vi "SDSU_ReadMux.vi"(7 "fd":i32, 8 "error in (no error)":errorcluster, 9 "argument":string, 10 "action":T3(ring), 11 "DACS":string[][](table)) -> (0 "error out":errorcluster, 1 "response":string, 2 "Table":string[][](table), 6 "fd out":i32)   [LabVIEW 2016]
panel:
  out "muxes out":T1(array[cluster])
  in  "muxes":T2
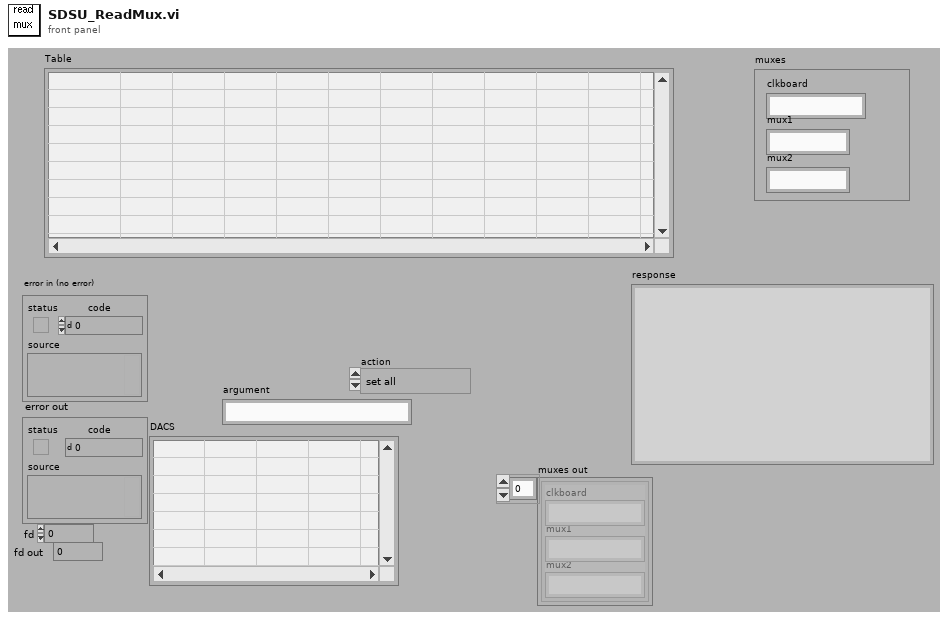
[diagram p1: front panel]
types:
  T1 = cluster{"clkboard":string, "mux1":string, "mux2":string}[]
  T2 = cluster{"clkboard":string, "mux1":string, "mux2":string}
  T3 = enum16{"set all", "set", "get all", "get list", "get"}
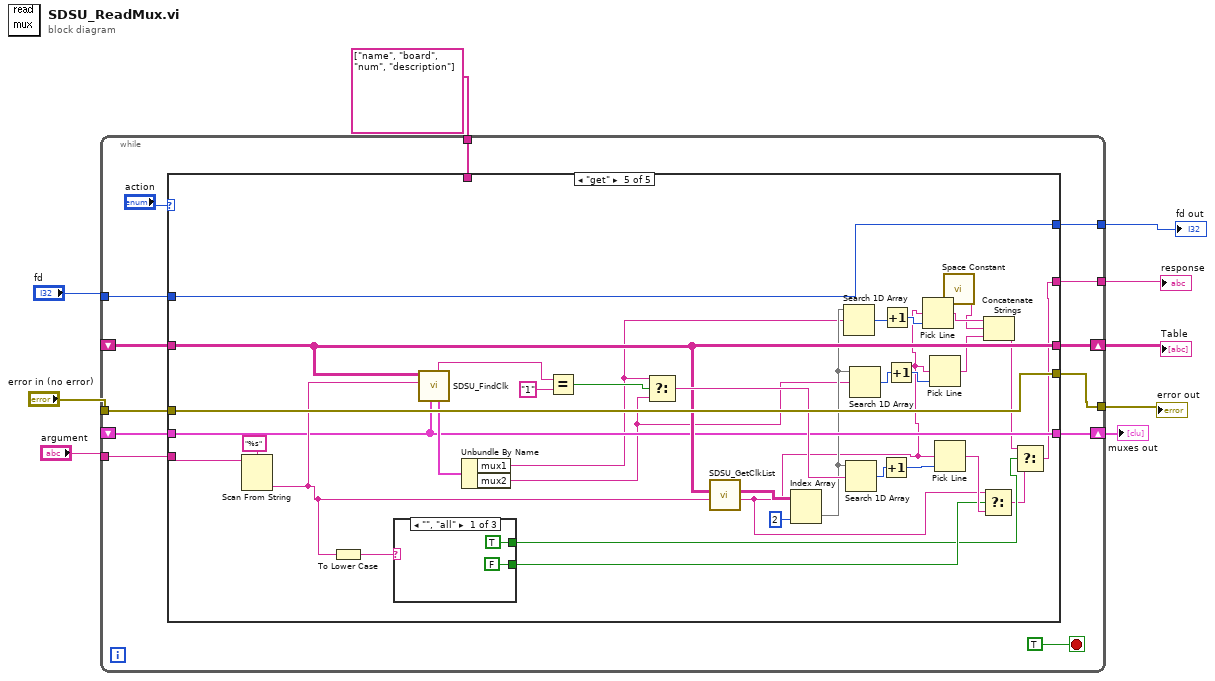
[diagram p0: block diagram]
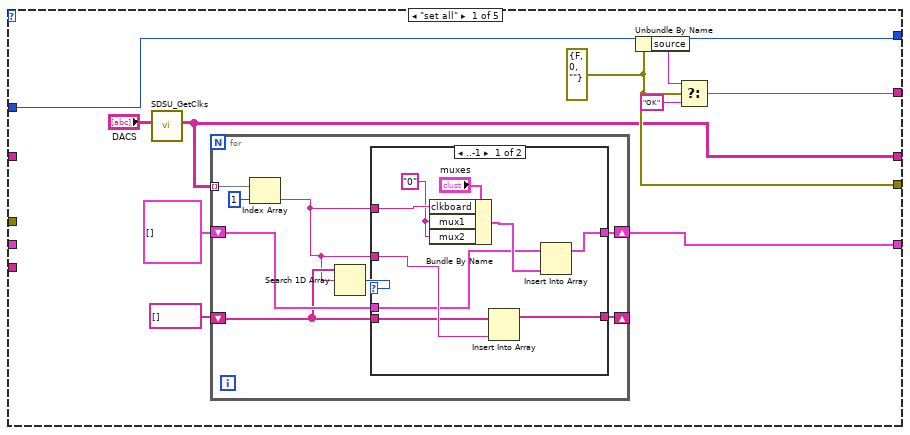
[diagram p2: hidden frame]
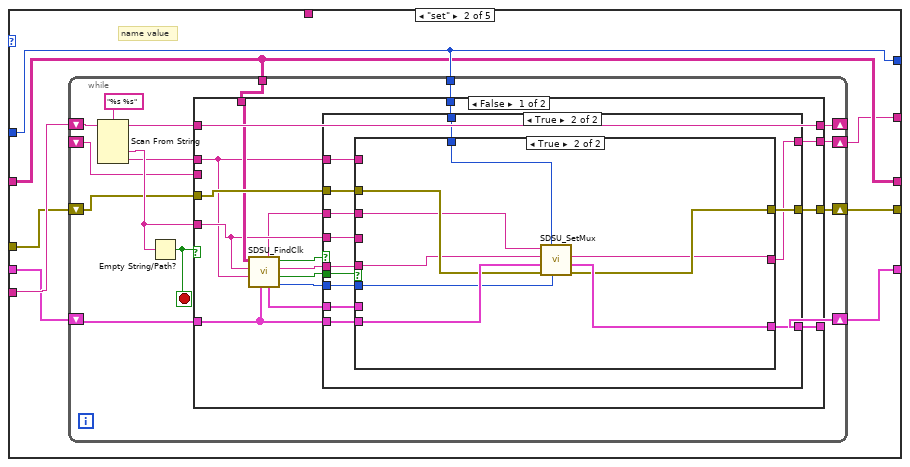
[diagram p4: hidden frame]
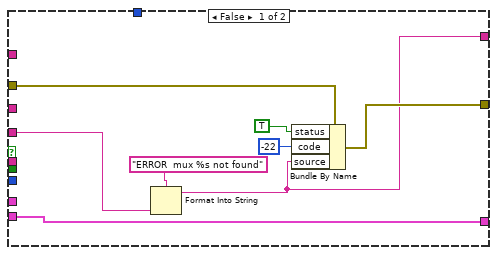
[diagram p5: hidden frame]
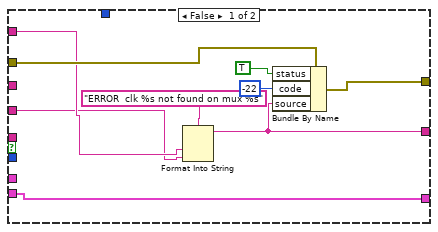
[diagram p6: hidden frame]
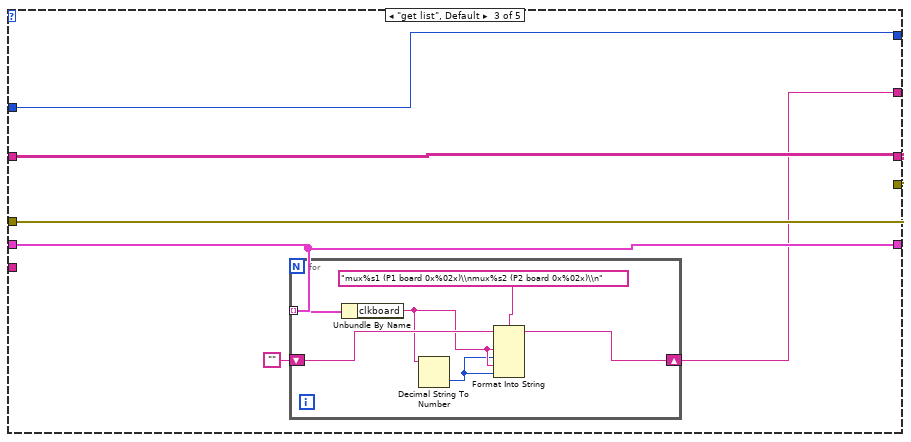
[diagram p8: hidden frame]
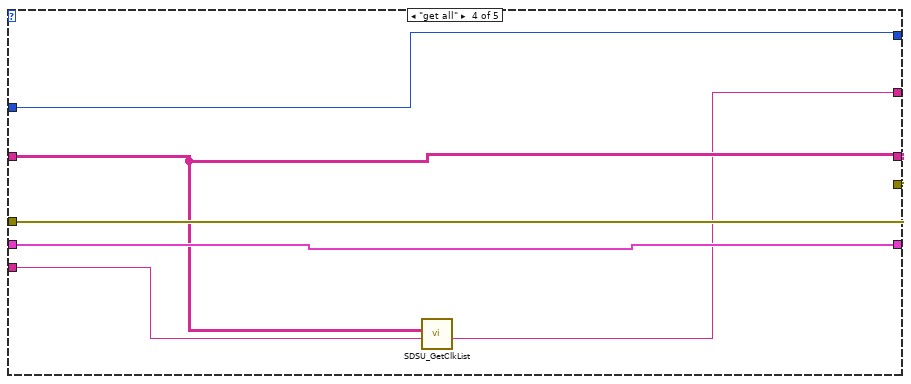
[diagram p9: hidden frame]
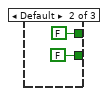
[diagram p10: hidden frame]
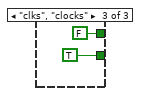
[diagram p11: hidden frame]
diagram:
  n1 = while {
    shift-right: [w21] -> w8
    shift-left: _ -> [w17]
    tunnel: "error in (no error)" -> [w20]
    tunnel: [w19] -> w2
    tunnel: [w10] -> w7
    tunnel: "argument" -> [w16]
    tunnel: "fd" -> [w15]
    tunnel: [w14] -> w4
    tunnel: string[] ["name", "board", "num", "description"] -> [w13]
    shift-right: [w12] -> w1
    shift-left: _ -> [w11]
    stop <- TRUE stop-if-true
    n2 = case shown="\"get\"" "action" {
      tunnel: [w27 w57 w137 w148 w168] -> w21
      tunnel: w20 -> [_ w53 w138 w150 w184]
      tunnel: [w28 w54 w138 w150 w184] -> w19
      tunnel: w17 -> [_ w57 w137 w148 w168]
      tunnel: w16 -> [_ w59 _ w147 w183]
      tunnel: w15 -> [w30 w58 w139 w151 w185]
      tunnel: [w30 w58 w139 w151 w185] -> w14
      tunnel: w13 -> [_ _ _ _ _]
      tunnel: [w26 w55 w136 w149 w167] -> w12
      tunnel: w11 -> [_ w56 w136 w149 w167]
      tunnel: [w23 w52 w134 w146 w152] -> w10
      frame "set all" {
        w28 = errorcluster {"status"=FALSE, "code"=0, "source"=""} ("input cluster")
        n3 = call "SDSU_GetClks.vi"("DACS"="DACS") -> ("Table"=w27:string[][])  [unwired: 10 out]
        n4 = for {
          tunnel: w27 -> [w40] mode=indexing
          shift-right: [w33] -> w26
          shift-left: T1 [] -> [w37]
          shift-right: [w36] -> _
          shift-left: string[] [] -> [w35]
          n5 = Index Array(array=w40, index=1) -> (element=w34:string)
          n6 = Search 1D Array(1D array=w35, element=w34) -> (index of element=w38:i32)  [unwired: 1 in]
          n7 = case shown="..-1" w38 {
            tunnel: w37 -> [w41 w50]
            tunnel: w34 -> [w49 _]
            tunnel: [w48 w51] -> w36
            tunnel: w35 -> [w47 w51]
            tunnel: w34 -> [w45 _]
            tunnel: [w42 w50] -> w33
            frame ..-1 {
              w44 = "0" ("element")
              n8 = Bundle By Name(cluster="muxes", "clkboard"=w45, "mux1"=w44, "mux2"=w44) -> (w43:T2)
              n9 = Insert Into Array(array=w47, new element=w49) -> (w48:string[])  [unwired: 1 in]
              n10 = Insert Into Array(array=w41, new element=w43) -> (w42:T1)  [unwired: 1 in]
            }
            frame Default {
            }
          }
        }
        n11 = Unbundle By Name(w28) -> ("source"=w32:string)
        n12 = Select(t=w32, s=w28, f="OK") -> (s? t:f=w23:string)
      }
      frame "set" {
        # "name value"
        n13 = while {
          shift-right: [w70] -> _
          shift-left: w59 -> [w73]
          tunnel: w58 -> [w67]
          tunnel: w57 -> [w66]
          shift-right: [w65] -> w55
          shift-left: w56 -> [w64]
          shift-right: [w63] -> w54
          shift-left: w53 -> [w62]
          shift-right: [w61] -> w52
          shift-left: _ -> [w60]
          stop <- w72 stop-if-true
          n14 = Scan From String(format string="%s %s", input string=w73) -> (remaining string=w71:string, output 1=w69:string, output 2=w68:string)  [unwired: 2 in, 4 out]
          n15 = Empty String/Path?(string/path=w69) -> (empty?=w72:bool)
          n16 = case shown="False" w72 {
            tunnel: w71 -> [w90 w133]
            tunnel: [w90 w133] -> w70
            tunnel: w69 -> [w84 _]
            tunnel: w62 -> [w89 w132]
            tunnel: w68 -> [w83 _]
            tunnel: [w88 w132] -> w63
            tunnel: [w87 w130] -> w61
            tunnel: w67 -> [w86 _]
            tunnel: w66 -> [w85 _]
            tunnel: w64 -> [w78 w131]
            tunnel: [w77 w131] -> w65
            tunnel: w60 -> [_ w130]
            frame False {
              n17 = call "SDSU_FindClk.vi"("muxes"=w78, "clk name"=w83, "mux name"=w84, "Table"=w85) -> ("mux index"=w75:i32, "found clk"=w81:bool, "clk num"=w80:string, "found mux"=w82:bool, "muxes out"=w79:T2, "mux num"=w76:string)  [unwired: 2 out]
              n18 = case shown="True" w82 {
                tunnel: w89 -> [w98 w110]
                tunnel: w84 -> [w94 w106]
                tunnel: [w93 w109] -> w88
                tunnel: [w92 w108] -> w87
                tunnel: w86 -> [_ w104]
                tunnel: w83 -> [_ w107]
                tunnel: w81 -> [_ w111]
                tunnel: w80 -> [_ w105]
                tunnel: w79 -> [_ w103]
                tunnel: w78 -> [w91 w102]
                tunnel: [w91 w100] -> w77
                tunnel: w76 -> [_ w101]
                tunnel: w75 -> [_ w99]
                frame False {
                  n19 = Format Into String(format string="ERROR  mux %s not found", w94) -> (resulting string=w92:string)  [unwired: 2 in, 1 out]
                  n20 = Bundle By Name(cluster=w98, "status"=TRUE, "code"=-22, "source"=w92) -> (w93:errorcluster)
                }
                frame True {
                  n21 = case shown="True" w111 {
                    tunnel: w110 -> [w118 w126]
                    tunnel: [w117 w127] -> w109
                    tunnel: [w116 w122] -> w108
                    tunnel: w107 -> [w113 _]
                    tunnel: w106 -> [w112 _]
                    tunnel: w105 -> [_ w124]
                    tunnel: w104 -> [_ w125]
                    tunnel: w103 -> [_ _]
                    tunnel: w102 -> [w114 w129]
                    tunnel: w101 -> [_ w121]
                    tunnel: [w114 w128] -> w100
                    tunnel: w99 -> [_ w123]
                    frame False {
                      n22 = Format Into String(format string="ERROR  clk %s not found on mux %s", w113, w112) -> (resulting string=w116:string)  [unwired: 2 in, 1 out]
                      n23 = Bundle By Name(cluster=w118, "status"=TRUE, "code"=-22, "source"=w116) -> (w117:errorcluster)
                    }
                    frame True {
                      n24 = call "SDSU_SetMux.vi"("muxes index"=w123, "fd"=w125, "error in (no error)"=w126, "muxes in"=w129, "clk"=w124, "mux"=w121) -> ("error IO"=w127:errorcluster, "muxes out"=w128:T1, "response"=w122:string)  [unwired: 3 out]
                    }
                  }
                }
              }
            }
            frame True {
            }
          }
        }
      }
      frame "get list", Default {
        n25 = for {
          tunnel: w136 -> [w142] mode=indexing
          shift-right: [w144] -> w134
          shift-left: "" -> [w143]
          n26 = Unbundle By Name(w142) -> ("clkboard"=w141:string)
          n27 = Decimal String To Number(string=w141) -> (number=w140:i32)  [unwired: 3 out]
          n28 = Format Into String(format string="mux%s1 (P1 board 0x%02x)\\nmux%s2 (P2 board 0x%02x)\\n", initial string=w143, w141, w140, w141, w140) -> (resulting string=w144:string)  [unwired: 1 in, 1 out]
        }
      }
      frame "get all" {
        n29 = call "SDSU_GetClkList.vi"("mux name"=w147, "Table"=w148) -> ("clks str"=w146:string)  [unwired: 9 out]
      }
      frame "get" {
        n30 = Scan From String(format string="%s", input string=w183) -> (output 1=w171:string)  [unwired: 2 in, 4 out]
        n31 = To Lower Case(string=w171) -> (all lower case string=w170:string)
        n32 = case shown="\"\", \"all\"" w170 {
          tunnel: [FALSE FALSE TRUE] -> w169
          tunnel: [TRUE FALSE FALSE] -> w155
          frame "", "all" {
          }
          frame Default {
          }
          frame "clks", "clocks" {
          }
        }
        n33 = call "SDSU_FindClk.vi"("muxes"=w167, "mux name"=w171, "Table"=w168) -> ("muxes out"=w181:T2, "mux num"=w180:string)  [unwired: 1 in, 6 out]
        n34 = Unbundle By Name(w181) -> ("mux1"=w165:string, "mux2"=w164:string)
        n35 = Equal?(x=w180, y="1") -> (x = y?=w178:bool)
        n36 = Select(t=w165, s=w178, f=w164) -> (s? t:f=w175:string)
        n37 = call "SDSU_GetClkList.vi"("mux name"=w171, "Table"=w168) -> ("clks str"=w156:string, "cloks"=w177:string[][])  [unwired: 8 out]
        n38 = Index Array(array=w177, index (col)=2 ("disabled index (col)")) -> (element=w166:string[])  [unwired: 1 in]
        n39 = Search 1D Array(1D array=w166, element=w165) -> (index of element=w163:i32)  [unwired: 1 out]
        n40 = Search 1D Array(1D array=w166, element=w175) -> (index of element=w174:i32)  [unwired: 1 out]
        n41 = Search 1D Array(1D array=w166, element=w164) -> (index of element=w162:i32)  [unwired: 1 out]
        n42 = Increment(x=w174) -> (x+1=w173:i32)
        n43 = Increment(x=w163) -> (x+1=w161:i32)
        n44 = Increment(x=w162) -> (x+1=w160:i32)
        n45 = Pick Line(multi-line string=w156, line index=w161) -> (output string=w159:string)  [unwired: 1 out]
        n46 = Pick Line(multi-line string=w156, line index=w160) -> (output string=w158:string)  [unwired: 1 out]
        n47 = Pick Line(multi-line string=w156, line index=w173) -> (output string=w172:string)  [unwired: 1 out]
        n48 = call <vilib>:"Space Constant.vi"() -> ("String"=w157:string)
        n49 = Select(t=w156, s=w169, f=w172) -> (s? t:f=w153:string)
        n50 = Concatenate Strings(w159, w157, w158) -> (w154:string)
        n51 = Select(t=w154, s=w155, f=w153) -> (s? t:f=w152:string)
      }
    }
  }
  "error out" <- w2
  "Table" <- w8
  "response" <- w7
  "fd out" <- w4
  "muxes out" <- w1
